vi "Down Shift Commanded.vi"(8 "error in":errorcluster) -> (0 "error out":errorcluster, 3 "Down Shift Commanded":bool)   [LabVIEW 2014]
uses:
  Global Objects.vi
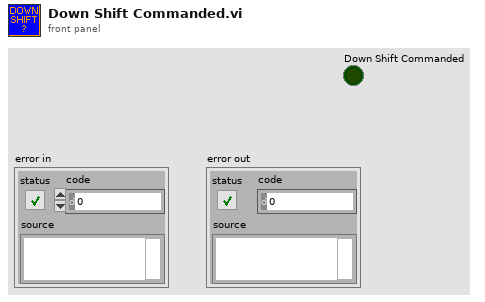
[diagram p1: front panel]
types:
  T1 = typedef "Teleop Commands.ctl" = cluster{"Throttle":dbl, "Turn":dbl, "Up Shift Commanded":bool, "Down Shift Commanded":bool}
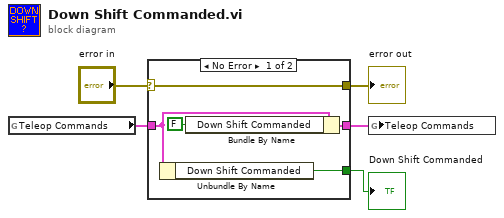
[diagram p0: block diagram]
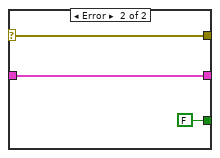
[diagram p2: hidden frame]
diagram:
  n1 = global read "Global Objects.vi" "Teleop Commands"() -> (w3:T1)
  n2 = case shown="No Error" "error in" {
    selector: "error in" -> [w9 w13]
    tunnel: [w9 w13] -> w4
    tunnel: [w7 w12] -> w2
    tunnel: w3 -> [w8 w12]
    tunnel: [w10 FALSE ("Up Shift Commanded")] -> w1
    frame No Error {
      n3 = Unbundle By Name(w8) -> ("Down Shift Commanded"=w10:bool)
      n4 = Bundle By Name(cluster=w8, "Down Shift Commanded"=FALSE ("Up Shift Commanded")) -> (w7:T1)
    }
    frame Error {
    }
  }
  "error out" <- w4
  "Down Shift Commanded" <- w1
  n5 = global write "Global Objects.vi" "Teleop Commands"(w2) -> ()
